vi "Test Get Named Range of Sheet (String).vi"(11 "Test Case In":refnum<class "Test Open Xml.lvclass">) -> (0 "error out":errorcluster, 3 "Test Case Out":refnum<class "Test Open Xml.lvclass">)   [LabVIEW 2021, in "Test Open Xml.lvclass"]
uses:
  Test Open Xml.lvclass
  C:/Program Files/National Instruments/LabVIEW 2025/vi.lib/Astemes/LUnit/Test Case.lvclass
  <vilib>/Astemes/LUnit/Test Case.lvclass/Test Case.ctl
  e7d09ce7-04db-40ce-9c4e-a78b31ec9fe8.vi
  <vilib>/Astemes/LUnit/Append Pass Result.vi
  <vilib>/Astemes/LUnit/Append Fail Result.vi
  e7d09ce7-04db-40ce-9c4e-a78b31ec9fe8.vi/9c5d11cd-9439-4240-a1ee-d9baace9c924.vi
  <vilib>/Astemes/LUnit/Run In UI.vi
  <vilib>/Utility/error.llb/Clear Errors.vi
  Source/Open Xml.lvlib
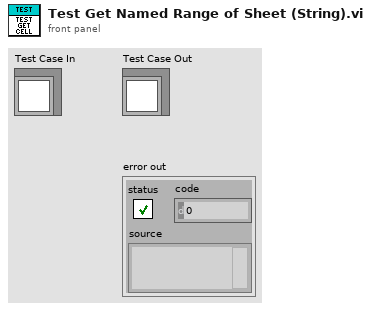
[diagram p1: front panel]
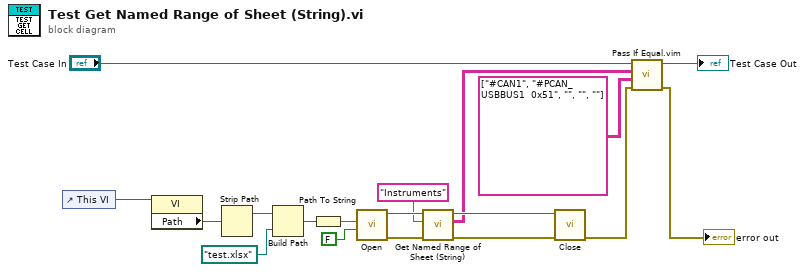
[diagram p0: block diagram]
diagram:
  n1 = control-ref of="This VI"() -> (w15:refnum<vi>)
  n2 = property class="VI"(reference=w15) -> ("Path"=w14:path)  [unwired: 1 in, 2 out]
  n3 = Strip Path(path=w14) -> (stripped path=w13:path)  [unwired: 1 out]
  n4 = Build Path(base path=w13, name or relative path=path "test.xlsx") -> (appended path=w11:path)
  n5 = Path To String(path=w11) -> (string=w10:string)
  n6 = call "Open.vi"("isEditable"=FALSE, "Path"=w10) -> ("error out"=w7:errorcluster, "SpreadsheetDocument"=w8:refnum<k24>)  [unwired: 8 in]
  n7 = call "Get Named Range of Sheet (String).vi"("error in"=w7, "Named Range Identifier"="Instruments" ("Sheet Name"), "SpreadsheetDocument"=w8) -> ("error out"=w5:errorcluster, "Cells"=w2:string[][], "SpreadsheetDocument out"=w3:refnum<k24>)  [unwired: 6 in]
  n8 = call "Close.vi"("error in"=w5, "SpreadsheetDocument"=w3) -> ("error out"=w4:errorcluster)  [unwired: 9 in]
  n9 = call "Pass If Equal.vim"("error in (no error)"=w4, "Actual"=string[][] [["#CAN1"], ["#PCAN_USBBUS1  0x51"], [""], [""], [""]] ("Cells"), "Expected"=w2, "LUnit Test Case In"="Test Case In") -> ("error out"=→"error out":errorcluster, "LUnit Test Case Out"=→"Test Case Out":refnum<class "Test Open Xml.lvclass">)  [unwired: 6 in]
